vi "Draw Title.vi"(9 "State Data":T2, 10 "Draw Area Size":T1, 11 "Margin":i16) -> (0 "mask":u8[](array[numeric]), 1 "24-bit pixmap":u32[][](array[numeric]), 2 "Draw Position":cluster{"x":i16, "y":i16}, 3 "Title Height":u32)   [LabVIEW 2018, in "PieChart.lvclass"]
uses:
  PieChart.lvclass
  <vilib>/Utility/miscctls.llb/LVFontTypeDef.ctl
  State Data.ctl
  <vilib>/Utility/miscctls.llb/LVBoundsTypeDef.ctl
  Pie info for Click.ctl
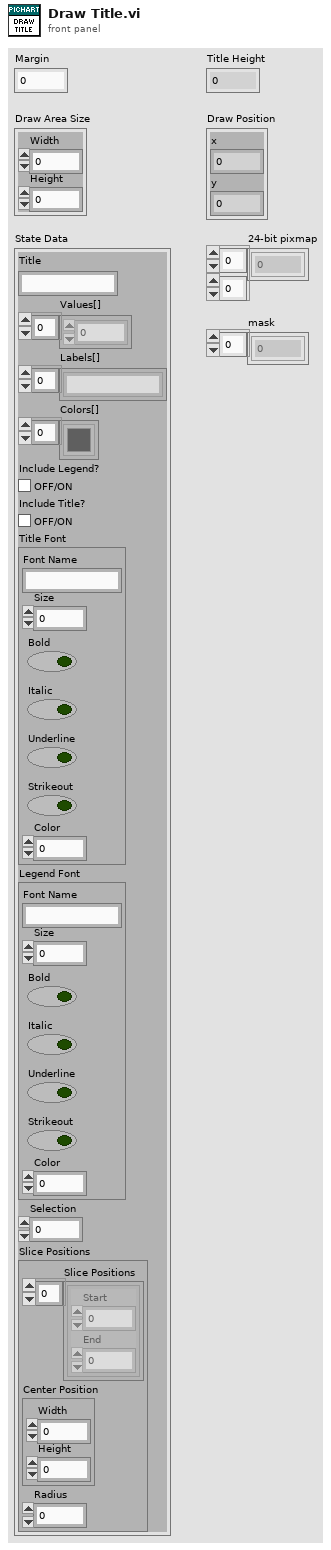
[diagram p1: front panel]
types:
  T1 = typedef "LVBoundsTypeDef.ctl" = cluster{"Width":u32, "Height":u32}
  T2 = typedef "PieChart.lvclass/State Data.ctl" = cluster{"Title":string, "Values[]":dbl[], "Labels[]":string[], "Colors[]":u32[], "Include Legend?":bool, "Include Title?":bool, "Title Font":T3, "Legend Font":T3, "Selection":i32, "Slice Positions":T4}
  T3 = typedef "LVFontTypeDef.ctl" = cluster{"Font Name":string, "Size":u16, "Bold":bool, "Italic":bool, "Underline":bool, "Strikeout":bool, "Color":u32}
  T4 = typedef "PieChart.lvclass/Pie info for Click.ctl" = cluster{"Slice Positions":cluster{"Start":i16, "End":i16}[], "Center Position":T1, "Radius":i16}
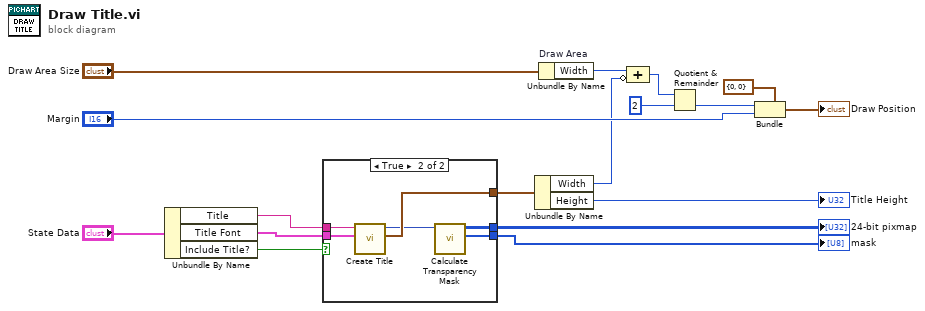
[diagram p0: block diagram]
diagram:
  n1 = Unbundle By Name("State Data") -> ("Title"=w17:string, "Title Font"=w16:T3, "Include Title?"=w15:bool)
  n2 = case shown="True" w15 {
    tunnel: w17 -> [_ w23]
    tunnel: w16 -> [_ w22]
    tunnel: [_ w21] -> w3
    tunnel: [_ w19] -> w8
    tunnel: [_ w18] -> w9
    frame False {
    }
    frame True {
      n3 = call "Create Title.vi"("Font"=w22, "Title"=w23) -> ("Title Box Size"=w21:cluster{"Width":u32, "Height":u32}, "Title out"=w20:picture)  [unwired: 8 in]
      n4 = call "Calculate Transparency Mask.vi"("Picture in"=w20) -> ("mask"=w18:u8[], "24-bit pixmap"=w19:u32[][])  [unwired: 8 in, 1 out]
    }
  }
  "mask" <- w9
  "24-bit pixmap" <- w8
  n5 = Unbundle By Name(w3) -> ("Width"=w1:u32, "Height"=→"Title Height":u32)
  n6 = Unbundle By Name "Draw Area"("Draw Area Size") -> ("Width"=w10:u32)
  n7 = Compound Arithmetic op=ADD(w10, invert w1) -> (w4:u32)
  n8 = Quotient & Remainder(x=w4, y=u32 2) -> (floor(x/y)=w6:u32)  [unwired: 1 out]
  n9 = Bundle(cluster=cluster{"x":i16, "y":i16} {"x"=0, "y"=0} ("top left point(0, 0)"), "x"=w6, "y"="Margin") -> (→"Draw Position":cluster{"x":i16, "y":i16})
